vi "Name.vi"(8 "error in (no error)":errorcluster, 11 "ReversiPlayer in":refnum<class "ReversiPlayer.lvclass">) -> (0 "error out":errorcluster, 2 "Name":string, 3 "ReversiPlayer out":refnum<class "ReversiPlayer.lvclass">)   [LabVIEW 2020, in "ReversiPlayer.lvclass"]
uses:
  ReversiPlayer.lvclass
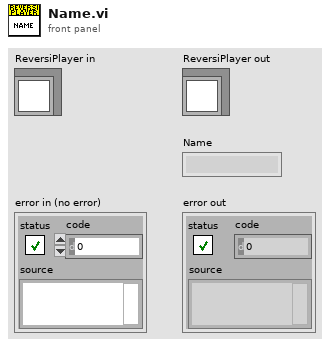
[diagram p1: front panel]
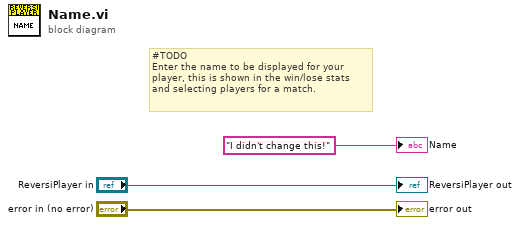
[diagram p0: block diagram]
diagram:
  # "#TODO\nEnter the name to be displayed for your player, this is shown in the win/lose stats and selecting players for a match."
  "error out" <- "error in (no error)"
  "ReversiPlayer out" <- "ReversiPlayer in"
  "Name" <- "I didn't change this!" ("Name")
